vi "Number Guesser.vi"() -> ()   [LabVIEW 2017]
panel:
  in  "Number to Match":u32 max=1000 step=1
  out "Numer of Iterations":dbl
  out "Current Number":u32
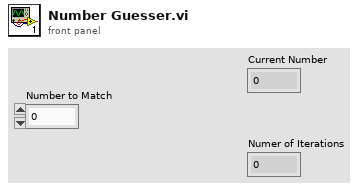
[diagram p1: front panel]
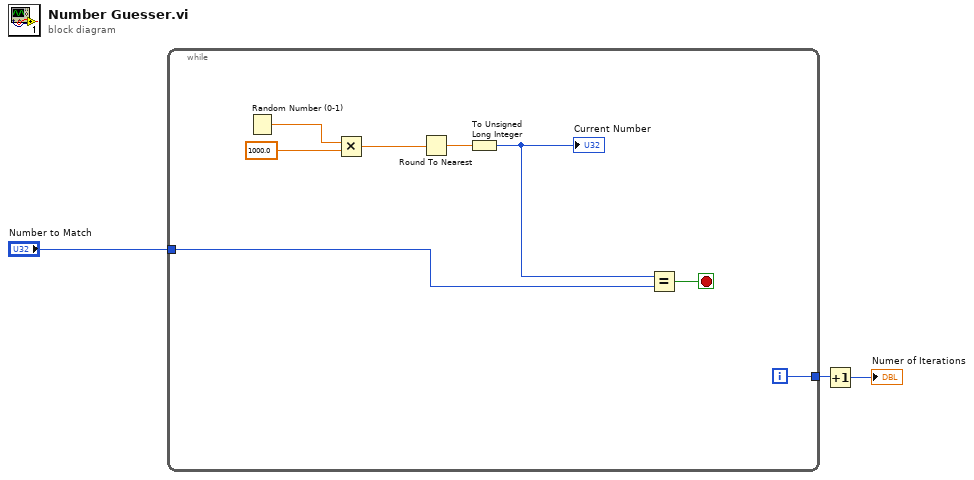
[diagram p0: block diagram]
diagram:
  n1 = while {
    tunnel: "Number to Match" -> [w7]
    tunnel: [w9] -> w1
    i -> [w9]
    stop <- w8 stop-if-true
    n2 = Random Number (0-1)() -> (number: 0 to 1=w10:dbl)
    n3 = Multiply(x=w10, y=1000.0 ("x*y")) -> (x*y=w6:dbl)
    n4 = Round To Nearest(number=w6) -> (nearest integer value=w5:dbl)
    n5 = To Unsigned Long Integer(number=w5) -> (unsigned 32bit integer=w4:u32)
    "Current Number" <- w4
    n6 = Equal?(x=w4, y=w7) -> (x = y?=w8:bool)
  }
  n7 = Increment(x=w1) -> (x+1=→"Numer of Iterations":i32)
